vi "Calibrate ADC Set Code.vi"(8 "error in":errorcluster, 9 "Gain Code":u16 format="%x", 10 "Input Channel":i32(ring) caption="Channel" items=["Input Channel 1", "Input Channel 2", "Input Channel 3", "Input Channel 4"], 11 "Instrument Handle In":i32) -> (0 "error out":errorcluster, 3 "Instrument Handle Out":i32)   [LabVIEW 8.6, in "ZTScopeM.lvlib"]
doc: "Set the instrument's ADC code setting for a specific channel. See the instrument calibration manual for more information."
uses:
  ZTScopeM.lvlib
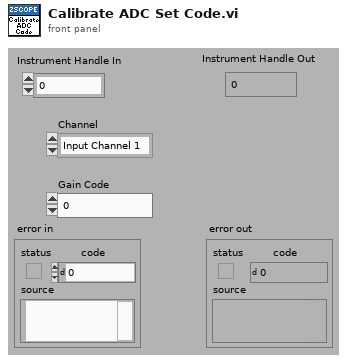
[diagram p1: front panel]
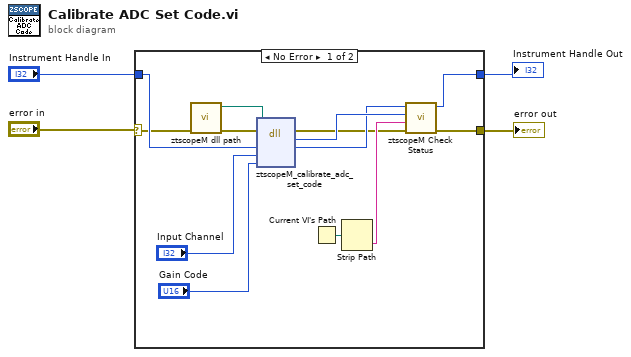
[diagram p0: block diagram]
diagram:
  n1 = case shown="No Error" "error in" {
    selector: "error in" -> [w8 w19]
    tunnel: [w12 w19] -> w1
    tunnel: "Instrument Handle In" -> [w17 w18]
    tunnel: [w11 w18] -> w3
    frame #0 {
      n2 = call "ztscopeM dll path.vi"("error in (no error)"=w8) -> ("error out"=w6:errorcluster, "<instrument>.dll path"=w7:path)  [unwired: 9 in]
      n3 = dll-call lib="C:/Program Files (x86)/National Instruments/LabVIEW 2013/instr.lib/ztscopem/ztscopeM.dll" fn="ztscopeM_calibrate_adc_set_code"(path in=w7, error in=w6, "instrumentHandle"=w17, "channel"="Input Channel", "gainCode"="Gain Code") -> (error out=w5:errorcluster, w14:i32, "instrumentHandle"=w13:i32)  [unwired: 3 in, 1 out]
      n4 = Current VI's Path() -> (path=w16:path)
      n5 = Strip Path(path=w16) -> (name=w15:string)  [unwired: 1 out]
      n6 = call "ztscopeM Check Status.vi"("error in"=w5, "name of VI"=w15, "status (return code)"=w14, "instrument handle in"=w13) -> ("error out"=w12:errorcluster, "instrument handle out"=w11:i32)  [unwired: 2 in]
    }
    frame #1 {
    }
  }
  "Instrument Handle Out" <- w3
  "error out" <- w1
